vi "Cartesian Manipulator Inertia (Trajectory).vi"(8 "error in (no error)":errorcluster, 10 "joint position trajectory":dbl[][](array[numeric]), 11 "serial arm in":refnum<class "NI_Robotics_Serial Robot Arm.lvclass">) -> (0 "error out":errorcluster, 2 "inertia matrix trajectory":dbl[][][](array[numeric]), 3 "serial arm out":refnum<class "NI_Robotics_Serial Robot Arm.lvclass">)   [LabVIEW 2017, in "NI_Kinematics.lvlib"]
doc: "Calculates a matrix that represents the kinetic energy of the end effector of a robotic arm in Cartesian space. Wire data to the <B>joint positions</B> input to determine the polymorphic instance to use or manually select the instance.\n\n<B>.m file:</B> cinertia"
uses:
  <vilib>/robotics/Kinematics/NI_Kinematics.lvlib
  <vilib>/robotics/Kinematics/Robot/NI_Robotics_Serial Robot Arm.lvclass
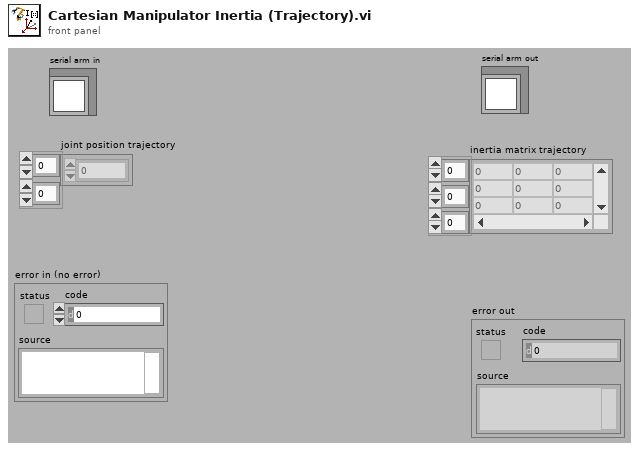
[diagram p1: front panel]
types:
  T1 = typedef "NI_Matrix.lvlib/RealMatrix.ctl" = dbl[][]
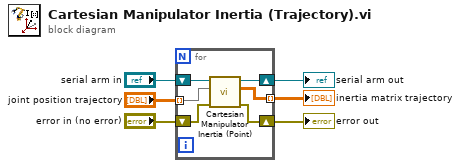
[diagram p0: block diagram]
diagram:
  n1 = for {
    tunnel: "joint position trajectory" -> [w12] mode=indexing
    tunnel: [w11] -> w5 mode=indexing
    shift-right: [w7] -> w1
    shift-left: "error in (no error)" -> [w8]
    shift-right: [w9] -> w3
    shift-left: "serial arm in" -> [w10]
    n2 = call <vilib>:"Cartesian Manipulator Inertia (Point).vi"("error in (no error)"=w8, "joint positions"=w12, "serial arm in"=w10) -> ("error out"=w7:errorcluster, "inertia matrix"=w11:T1, "serial arm out"=w9:refnum<class "NI_Robotics_Serial Robot Arm.lvclass">)  [unwired: 6 in]
  }
  "serial arm out" <- w3
  "inertia matrix trajectory" <- w5
  "error out" <- w1
